vi "drag Markers.vi"(6 "Marker Options":T1={"Color"=16723218, "Text"="Drag and click to position a marker", "Type"=enum."point", "pen"={"Width"=2, "Style"=enum."Solid"}, "font"={"Font Name"="Arial", "Size"=16, "Strikeout?"=FALSE, "Italic?"=FALSE, "Underline?"=FALSE, "Outline?"=FALSE, "Shadow?"=FALSE, "Bold?"=FALSE, "Color Box"=0}}, 8 "Error In":errorcluster, 10 "Coords":T2, 11 "XYGraph in":refnum<vi>) -> (0 "Error Out":errorcluster, 3 "new picture":picture)   [LabVIEW 2015]
doc: "Draw notes overlayed on the grph using picture control elements in the graph. This draws a line at the mouse location."
uses:
  <vilib>/Utility/miscctls.llb/LVPoint32TypeDef.ctl
  controls/AnnotationOptions.ctl
panel:
  in  "picture":picture
  out "XYGraph out":refnum<vi>
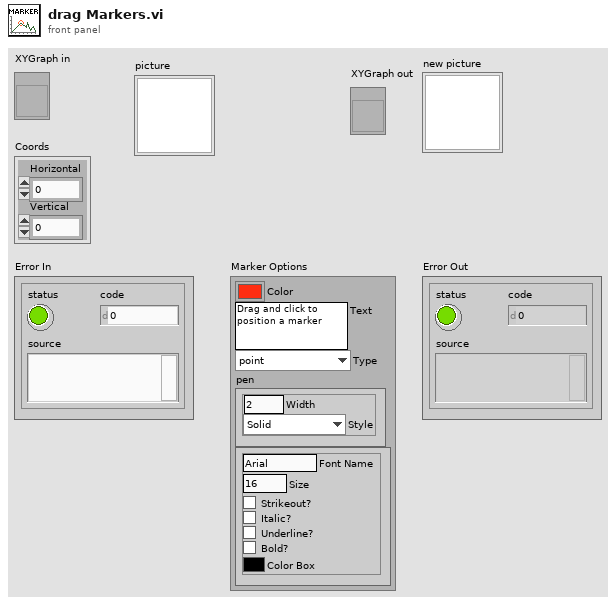
[diagram p1: front panel]
types:
  T1 = typedef "AnnotationOptions.ctl" = cluster{"Color":u32, "Text":string, "Type":enum16{"point", "horiz", "vert", "vert range", "horiz range", "box"}, "pen":cluster{"Width":u16, "Style":enum32{"Solid", "Dash", "Dot", "DashDot", "DashDotDot"}}, "font":cluster{"Font Name":string, "Size":i16, "Strikeout?":bool, "Italic?":bool, "Underline?":bool, "Outline?":bool, "Shadow?":bool, "Bold?":bool, "Color Box":u32}}
  T2 = typedef "LVPoint32TypeDef.ctl" = cluster{"Horizontal":i32, "Vertical":i32}
  T3 = typedef "LVRectTypeDef.ctl" = cluster{"Left":i16, "Top":i16, "Right":i16, "Bottom":i16}
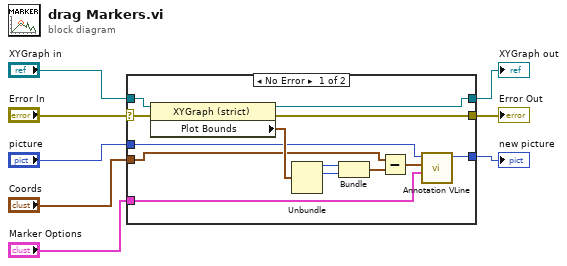
[diagram p0: block diagram]
diagram:
  n1 = case shown="No Error" "Error In" {
    selector: "Error In" -> [w18 w24]
    tunnel: "XYGraph in" -> [w20 w23]
    tunnel: "Coords" -> [w14 _]
    tunnel: [w19 w24] -> w5
    tunnel: [w21 w23] -> w4
    tunnel: "Marker Options" -> [w9 _]
    tunnel: "picture" -> [w11 w22]
    tunnel: [w10 w22] -> w1
    frame No Error {
      n2 = property on="Property Node" class="XYGraph (strict)"(reference=w20, error in=w18) -> (reference out=w21:refnum<vi>, error out=w19:errorcluster, "Plot Bounds"=w15:T3)
      n3 = Unbundle(w15) -> ("Left"=w16:i16, "Top"=w17:i16)  [unwired: 2 out]
      n4 = Bundle("Left"=w16, "Top"=w17) -> (w13:cluster{"Left":i16, "Top":i16})  [unwired: 1 in]
      n5 = Subtract(x=w14, y=w13) -> (x-y=w12:T2)
      n6 = call "Annotation VLine.vi"("Marker Options"=w9, "position"=w12, "picture"=w11) -> ("new picture"=w10:picture)  [unwired: 8 in]
    }
    frame Error {
    }
  }
  "Error Out" <- w5
  "XYGraph out" <- w4
  "new picture" <- w1
